vi "Beam_Check_Positions.vi"(1 "Values":dbl[][](array[numeric]) format="%.4f", 3 "Mode":T2(ring)) -> (0 "Values Out":dbl[][](array[numeric]) format="%.2f")   [LabVIEW 2010]
uses:
  Controls/Beam_Type.ctl
  Globals/Constants_global.vi
  Globals/Trav_pos_global.vi
panel:
  in  "Beam Type":T1 items=["Green Unshifted", "Green Shifted", "Blue Unshifted", "Blue Shifted"]
  # "X                                  Y                          Z             Datum Power"
  # "X                    Y                 Z"
  # "Green Unshifted\nGreen Shifted\nBlue Unshifted\nBlue Shifted"
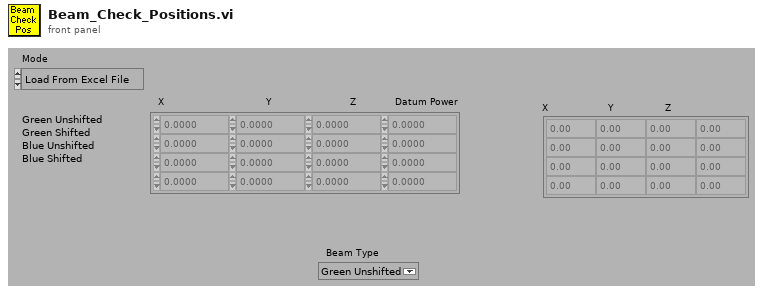
[diagram p1: front panel]
types:
  T1 = typedef "Beam_Type.ctl" = u16
  T2 = enum16{"Load From Excel File", "Save to Excel File"}
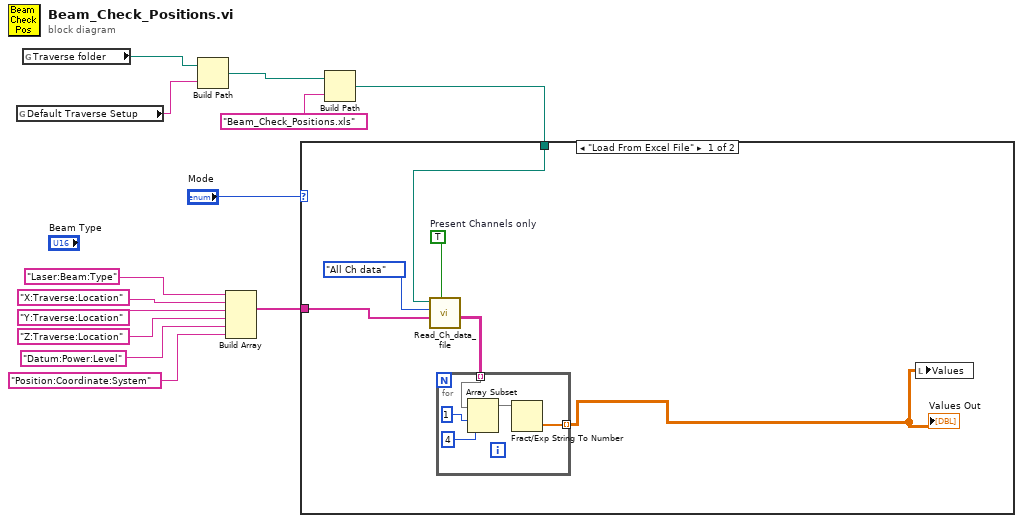
[diagram p0: block diagram]
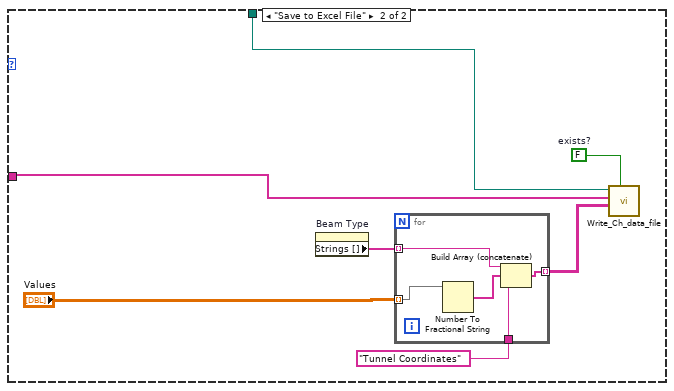
[diagram p2: hidden frame]
diagram:
  n1 = global read "Trav_pos_global.vi" "Default Traverse Setup"() -> (w2:string)
  n2 = global read "Constants_global.vi" "Traverse folder"() -> (w9:path)
  n3 = Build Path(base path=w9, name or relative path=w2) -> (appended path=w4:path)
  n4 = Build Array("Laser:Beam:Type", "X:Traverse:Location", "Y:Traverse:Location", "Z:Traverse:Location", "Datum:Power:Level", "Position:Coordinate:System") -> (w8:string[])
  n5 = Build Path(base path=w4, name or relative path="Beam_Check_Positions.xls" ("Substring")) -> (appended path=w3:path)
  n6 = case shown="\"Load From Excel File\"" "Mode" {
    tunnel: w8 -> [w17 w29]
    tunnel: w3 -> [w16 w30]
    frame "Load From Excel File" {
      w19 = TRUE  # Present Channels only
      n7 = call "Read_Ch_data_file.vi"("Present Channels only"=w19, "Present Channels"=w17, "Output"=enum16{"All Ch data", "The last few rows"}."All Ch data", "Filename"=w16) -> ("Channel Values"=w15:string[][])  [unwired: 1 in, 4 out]
      n8 = for {
        tunnel: w15 -> [w23] mode=indexing
        tunnel: [w21] -> w14 mode=indexing
        n9 = Array Subset(array=w23, index=1 ("Array Index"), length=4) -> (w22:string[])
        n10 = Fract/Exp String To Number(string=w22) -> (number=w21:dbl[])  [unwired: 4 out]
      }
      "Values Out" <- w14
      n11 = local write "Values"(w14) -> ()
    }
    frame "Save to Excel File" {
      w31 = FALSE  # exists?
      n12 = property on="Beam Type" class="Ring (strict)"() -> ("Strings []"=w28:string[])  [unwired: 2 in, 2 out]
      n13 = for {
        tunnel: "Values" -> [w36] mode=indexing
        tunnel: w28 -> [w35] mode=indexing
        tunnel: [w33] -> w27 mode=indexing
        tunnel: "Tunnel Coordinates" -> [w32]
        n14 = Number To Fractional String(number=w36) -> (F-format string=w34:string[])  [unwired: 3 out]
        n15 = Build Array (concatenate)(w35, w34, w32) -> (w33:string[])
      }
      n16 = call "Write_Ch_data_file.vi"("exists?"=w31, "Channel Values"=w27, "Channel names"=w29, "Filename"=w30) -> ()  [unwired: 4 in, 4 out]
    }
  }
